vi "ExFileReadNDisplayRGBGainOffset.vi"() -> ()   [LabVIEW 2010]
panel:
  out "Blue Offset":dbl format="%.2f"
  out "Green Offset":dbl format="%.2f"
  out "Red Offset":dbl format="%.2f"
  out "Blue Gain":dbl format="%.2f"
  out "Green Gain":dbl format="%.2f"
  out "Red Gain":dbl format="%.2f"
  in  "Blue Offset":dbl format="%.2f"
  in  "Green Offset":dbl format="%.2f"
  in  "Red Offset":dbl format="%.2f"
  in  "Blue Gain":dbl=1.0 format="%.2f"
  in  "Red Gain":dbl=1.0 format="%.2f"
  in  "Green Gain":dbl=1.0 format="%.2f"
  in  "Bit shift":u16
  in  "Type of Bayer":u32=1 max=1 step=1
  in  "Full File Name":path
  in  "?":bool
  in  "FileType":u32=67371008
  out "error out":errorcluster
  in  "error in (no error)":errorcluster
  # "ExReadFileNDisplayRGB.vi\nThis example will read in a file of the\nselected data type and display as RGB frame.\nWhen finished viewing data, make sure to\nuse the STOP button to close the display."
  # "File Types:\nSPE = 67371008\nTIF   = 67174400\nPMI  = 67436544"
  # "This will properly close\nthe image and\ndeallocate memory."
  # "Browse match pattern is set to *.spe.  Modify this if different file type is needed."
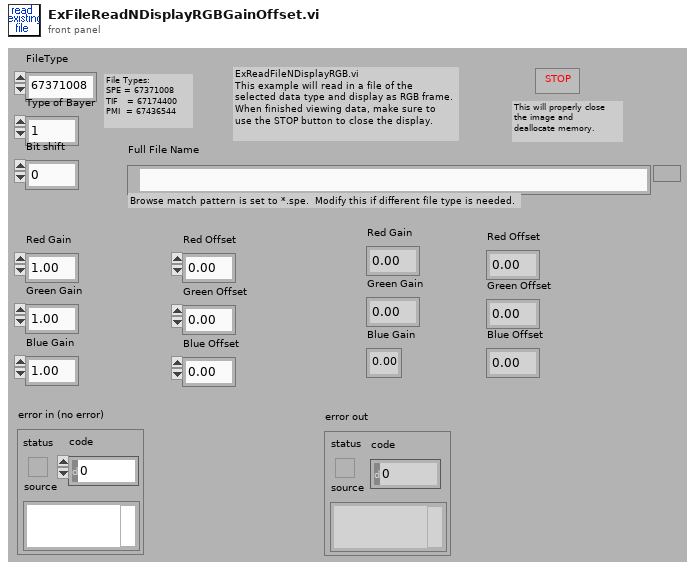
[diagram p1: front panel]
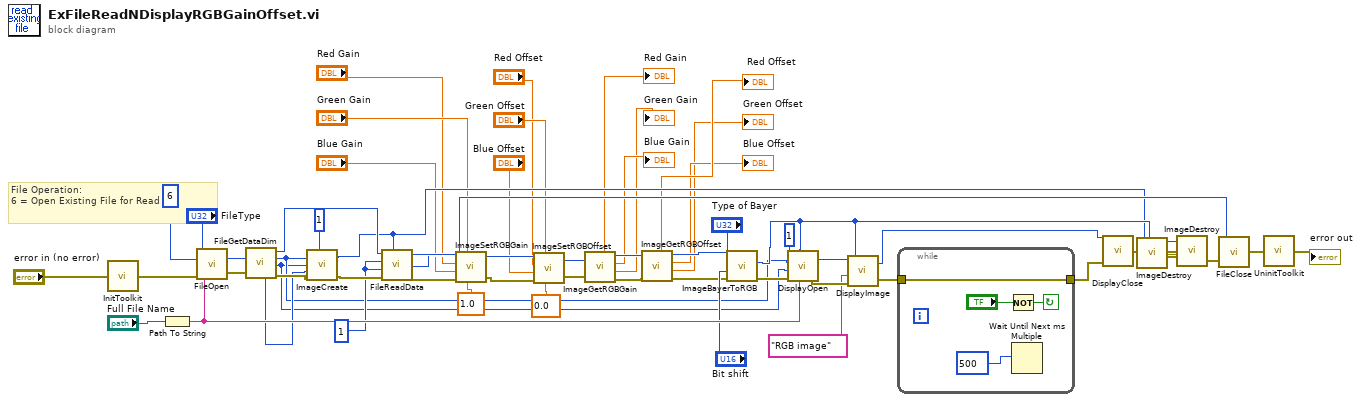
[diagram p0: block diagram]
diagram:
  w40 = 1
  # "File Operation:\n6 = Open Existing File for Read"
  n1 = call <userlib>:"InitToolkit.vi"("error in"="error in (no error)") -> ("error out"=w56:errorcluster)
  n2 = Path To String(path="Full File Name") -> (string=w45:string)
  n3 = call <userlib>:"FileOpen.vi"("error in"=w56, "File Operations"=u32 6 ("File Operation"), "FileName"=w45, "File Type"="FileType") -> ("error out"=w54:errorcluster, "File Handle"=w53:u32)
  n4 = call <userlib>:"FileGetDataDim.vi"("File Handle"=w53, "error in"=w54) -> ("Data Type"=w28:u32, "File Handle"=w42:u32, "X dim"=w2:u32, "Y dim"=w1:u32, "error out"=w52:errorcluster)  [unwired: 1 out]
  n5 = call <userlib>:"ImageCreate.vi"("X dimension"=w2, "Y dimension"=w1, "Data Type"=w28, "error in"=w52, "Number Of Frames"=1) -> ("Image Handle"=w31:u32, "error out"=w41:errorcluster)
  n6 = call <userlib>:"FileReadData.vi"("File Handle"=w42, "Start Frame"=w40, "End Frame"=w40, "error in"=w41, "Image Handle"=w31) -> ("File Handle"=w39:u32, "Image Handle"=w26:u32, "error out"=w25:errorcluster)
  n7 = call <userlib>:"ImageSetRGBGain.vi"("reserved"=1.0, "Green Gain"="Green Gain", "error in (no error)"=w25, "Blue Gain"="Blue Gain", "Red Gain"="Red Gain", "Image Handle"=w26) -> ("error out"=w23:errorcluster, "Image Handle"=w24:u32)
  n8 = call <userlib>:"ImageSetRGBOffset.vi"("reserved"=0.0, "Green Offset"="Green Offset", "error in (no error)"=w23, "Blue Offset"="Blue Offset", "Red Offset"="Red Offset", "Image Handle"=w24) -> ("error out"=w14:errorcluster, "Image Handle"=w9:u32)
  n9 = call <userlib>:"ImageGetRGBGain.vi"("Image Handle"=w9, "error in (no error)"=w14) -> ("Red"=→"Red Gain":dbl, "Image Handle"=w10:u32, "Blue"=→"Blue Gain":dbl, "Green"=→"Green Gain":dbl, "error out"=w13:errorcluster)  [unwired: 1 out]
  n10 = call <userlib>:"ImageGetRGBOffset.vi"("Image Handle"=w10, "error in (no error)"=w13) -> ("Red"=→"Red Offset":dbl, "Image Handle"=w11:u32, "Blue"=→"Blue Offset":dbl, "Green"=→"Green Offset":dbl, "error out"=w12:errorcluster)  [unwired: 1 out]
  n11 = call <userlib>:"ImageBayerToRGB.vi"("Image Handle"=w11, "Type of Bayer"="Type of Bayer", "Shift amount"="Bit shift", "error in"=w12) -> ("RGB Image Handle"=w32:u32, "error out"=w44:errorcluster)  [unwired: 1 in, 1 out]
  n12 = call <userlib>:"DisplayOpen.vi"("Display Title"=w45, "Image Handle"=w32, "error in"=w44, "Display Height"=w1, "Display Width"=w2, "Display Type"=1) -> ("error out"=w38:errorcluster, "Display Handle"=w37:u32)
  n13 = call <userlib>:"DisplayImage.vi"("error in"=w38, "Title"="RGB image", "Image Handle"=w32, "Display Handle"=w37) -> ("error out"=w30:errorcluster, "Display Handle"=w36:u32)
  n14 = while {
    tunnel: w30 -> [w59]
    tunnel: [w59] -> w29
    stop <- w61 continue-if-true
    n15 = Not(x="?") -> (.not. x?=w61:bool)
    n16 = Wait Until Next ms Multiple(millisecond multiple=500) -> ()  [unwired: 1 out]
  }
  n17 = call <userlib>:"DisplayClose.vi"("error in"=w29, "Display Handle"=w36) -> ("error out"=w49:errorcluster)
  n18 = call <userlib>:"ImageDestroy.vi"("error in"=w49, "Data handle"=w32) -> ("error out"=w35:errorcluster)
  n19 = call <userlib>:"ImageDestroy.vi"("error in"=w35, "Data handle"=w31) -> ("error out"=w34:errorcluster)
  n20 = call <userlib>:"FileClose.vi"("error in"=w34, "File Handle"=w39) -> ("error out"=w48:errorcluster)
  n21 = call <userlib>:"UninitToolkit.vi"("error in"=w48) -> ("error out"=→"error out":errorcluster)
